vi "Shutdown Plugin Subpanel Events.vi"(8 "error in (no error)":errorcluster, 11 "CIF_UI in":refnum<class "CIF_UI.lvclass">) -> (0 "error out":errorcluster)   [LabVIEW 2021, in "CIF_UI.lvclass"]
uses:
  CIF_UI.lvclass
  CIF_UI.lvclass/CIF_UI.ctl
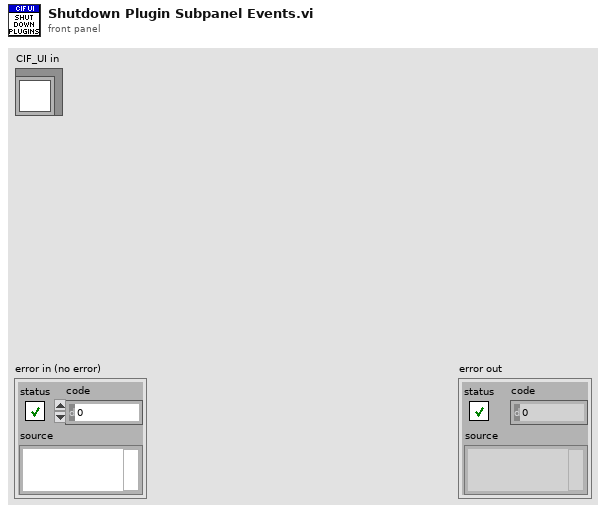
[diagram p1: front panel]
types:
  T1 = typedef "CIF_UI.lvclass/Plugin Subpanel Map.ctl" = map{i32, T2}
  T2 = typedef "CIF_UI.lvclass/Subpanel Data.ctl" = cluster{"VI Reference":refnum<vi>, "Plugin Subpanel Events":T3}
  T3 = typedef "CIF_UI.lvclass/Plugin Subpanel Events.ctl" = cluster{"Plugin Shutdown":refnum<user-event>}
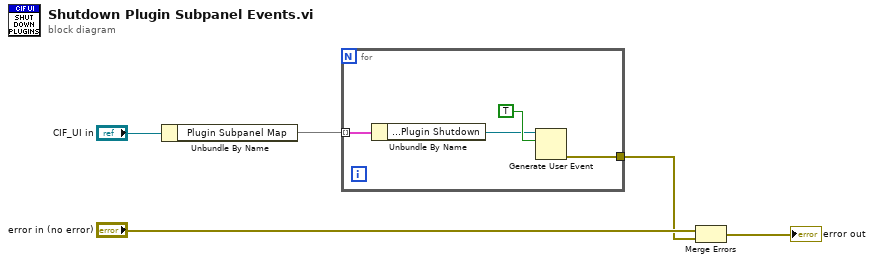
[diagram p0: block diagram]
diagram:
  n1 = Unbundle By Name("CIF_UI in") -> ("Plugin Subpanel Map"=w4:T1)
  n2 = for {
    tunnel: w4 -> [w7] mode=indexing
    tunnel: [w8] -> w2
    n3 = Unbundle By Name(w7) -> ("SubPanel Data.Plugin Subpanel Events.Plugin Shutdown"=w6:refnum<user-event>)
    n4 = Generate User Event(user event=w6, event data cluster=TRUE ("event data")) -> (error out=w8:errorcluster)  [unwired: 2 in, 1 out]
  }
  n5 = Merge Errors("error in (no error)", w2) -> (→"error out":errorcluster)
